vi "Fully Dynamic FPGA Interface Example.vi"() -> ()   [LabVIEW 2010]
uses:
  <vilib>/userDefined/High Color/nirio_resource_hc.ctl
  TypeDefs/Fully Dynamic FPGA Interface TypeDef.ctl
  <vilib>/Utility/sysdir.llb/System Directory Type.ctl
  <userlib>/_FPGA Interface Advanced Tools/FPGA Interface Base/FPGA Interface Base.lvclass
  <userlib>/_FPGA Interface Advanced Tools/FPGA Bitfile Utility/Get Register Map.vi
  <userlib>/_FPGA Interface Advanced Tools/FPGA Bitfile Utility/Get Base Address.vi
  <vilib>/rvi/Utilities/XML/nirviXML_GetValue.vi
  <vilib>/rvi/Utilities/XML/nirviXML_GetValue_String.vi
  <vilib>/rvi/Bitfile/niFpgaReadBitfileXml_VIRegisterMap.vi
  <vilib>/rvi/Utilities/XML/nirviXML_GetValue_U32.vi
  <vilib>/Utility/VariantDataType/GetTypeInfo.vi
  <vilib>/Utility/VariantDataType/GetArrayInfo.vi
  <userlib>/_FPGA Interface Advanced Tools/FPGA Interface Base/FPGA Read By Name - Boolean.vi
  <userlib>/_FPGA Interface Advanced Tools/FPGA Interface Base/FPGA Read By Name - I8.vi
  <userlib>/_FPGA Interface Advanced Tools/FPGA Interface Base/FPGA Read By Name - I16.vi
  <userlib>/_FPGA Interface Advanced Tools/FPGA Interface Base/FPGA Read By Name - I32.vi
  <userlib>/_FPGA Interface Advanced Tools/FPGA Interface Base/FPGA Read By Name - I64.vi
  <userlib>/_FPGA Interface Advanced Tools/FPGA Interface Base/FPGA Read By Name - U8.vi
  <userlib>/_FPGA Interface Advanced Tools/FPGA Interface Base/FPGA Read By Name - U16.vi
  <userlib>/_FPGA Interface Advanced Tools/FPGA Interface Base/FPGA Read By Name - U32.vi
  <userlib>/_FPGA Interface Advanced Tools/FPGA Interface Base/FPGA Read By Name - U64.vi
  <userlib>/_FPGA Interface Advanced Tools/FPGA Interface Base/FPGA Read Array By Name - Boolean.vi
  <userlib>/_FPGA Interface Advanced Tools/FPGA Interface Base/FPGA Read Array By Name - I8.vi
  <userlib>/_FPGA Interface Advanced Tools/FPGA Interface Base/FPGA Read Array By Name - I16.vi
  <userlib>/_FPGA Interface Advanced Tools/FPGA Interface Base/FPGA Read Array By Name - I32.vi
  <userlib>/_FPGA Interface Advanced Tools/FPGA Interface Base/FPGA Read Array By Name - I64.vi
  <userlib>/_FPGA Interface Advanced Tools/FPGA Interface Base/FPGA Read Array By Name - U8.vi
  <userlib>/_FPGA Interface Advanced Tools/FPGA Interface Base/FPGA Read Array By Name - U16.vi
  <userlib>/_FPGA Interface Advanced Tools/FPGA Interface Base/FPGA Read Array By Name - U32.vi
  <userlib>/_FPGA Interface Advanced Tools/FPGA Interface Base/FPGA Read Array By Name - U64.vi
  <userlib>/_FPGA Interface Advanced Tools/FPGA Interface Base/FPGA Write By Name - Boolean.vi
  <userlib>/_FPGA Interface Advanced Tools/FPGA Interface Base/FPGA Write By Name - I8.vi
  <userlib>/_FPGA Interface Advanced Tools/FPGA Interface Base/FPGA Write By Name - I16.vi
  <userlib>/_FPGA Interface Advanced Tools/FPGA Interface Base/FPGA Write By Name - I32.vi
  <userlib>/_FPGA Interface Advanced Tools/FPGA Interface Base/FPGA Write By Name - I64.vi
  <userlib>/_FPGA Interface Advanced Tools/FPGA Interface Base/FPGA Write By Name - U8.vi
  <userlib>/_FPGA Interface Advanced Tools/FPGA Interface Base/FPGA Write By Name - U16.vi
  <userlib>/_FPGA Interface Advanced Tools/FPGA Interface Base/FPGA Write By Name - U32.vi
  <userlib>/_FPGA Interface Advanced Tools/FPGA Interface Base/FPGA Write By Name - U64.vi
  <userlib>/_FPGA Interface Advanced Tools/FPGA Interface Base/FPGA Write Array By Name - Boolean.vi
  <userlib>/_FPGA Interface Advanced Tools/FPGA Interface Base/FPGA Write Array By Name - I8.vi
  <userlib>/_FPGA Interface Advanced Tools/FPGA Interface Base/FPGA Write Array By Name - I16.vi
  <userlib>/_FPGA Interface Advanced Tools/FPGA Interface Base/FPGA Write Array By Name - I32.vi
  <userlib>/_FPGA Interface Advanced Tools/FPGA Interface Base/FPGA Write Array By Name - I64.vi
  <userlib>/_FPGA Interface Advanced Tools/FPGA Interface Base/FPGA Write Array By Name - U8.vi
  <userlib>/_FPGA Interface Advanced Tools/FPGA Interface Base/FPGA Write Array By Name - U16.vi
  <userlib>/_FPGA Interface Advanced Tools/FPGA Interface Base/FPGA Write Array By Name - U32.vi
  <userlib>/_FPGA Interface Advanced Tools/FPGA Interface Base/FPGA Write Array By Name - U64.vi
  <userlib>/_FPGA Interface Advanced Tools/FPGA Bitfile Utility/FPGA Bitfile Utility.lvlib
panel:
  in  "RIO Resource":T1="RIO0"
  out "Boolean Array Read":bool[](array[boolean])
  in  "Boolean Array Write":bool[](array[boolean])
  in  "Numeric Array Write":dbl[](array[numeric])
  out "Numeric Array Read":dbl[](array[numeric])
  in  "Numeric Write":dbl
  out "Numeric Read":dbl
  in  "Boolean Write":bool
  out "Bool Read":bool
  in  "Write":bool
  in  "Read":bool
  in  "Multicolumn Listbox":i32(listbox)
  in  "Stop FPGA":bool
  in  "Run FPGA":bool
  in  "Select Bitfile":bool
  out "Bifile Path":path
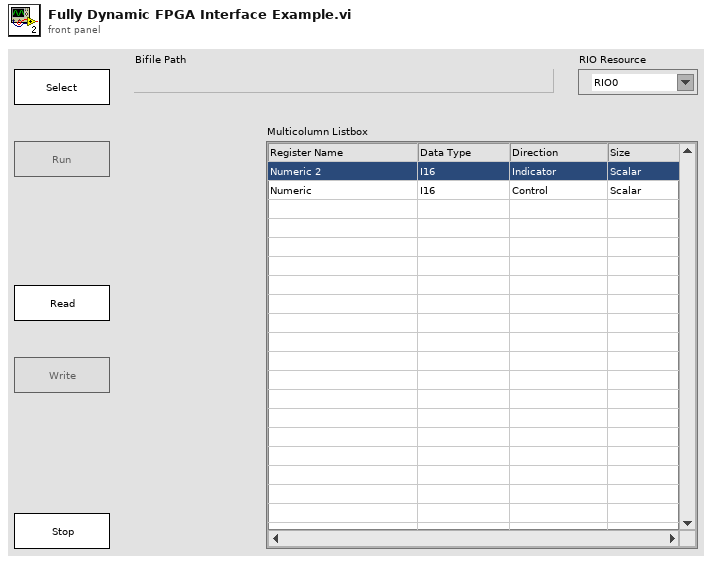
[diagram p1: front panel]
types:
  T1 = typedef "nirio_resource_hc.ctl" = tag
  T2 = typedef "Fully Dynamic FPGA Interface TypeDef.ctl" = enum16{"Idle", "Init", "Read", "Write"}
  T3 = enum8{"Enabled", "Disabled", "Disabled and Grayed Out"}
  T4 = typedef "System Directory Type.ctl" = i32
  T5 = typedef "FPGA Bitfile Utility.lvlib/Control_Indicator Info.ctl" = cluster{"Array?":bool, "Data Type":T6, "Address":u32, "Num Elements":u32, "Name":string}
  T6 = typedef "niFpgaDataTypeControl.ctl" = enum32{"Boolean", "I8", "I16", "I32", "I64", "U8", "U16", "U32", "U64", "FXP", "CustomControl"}
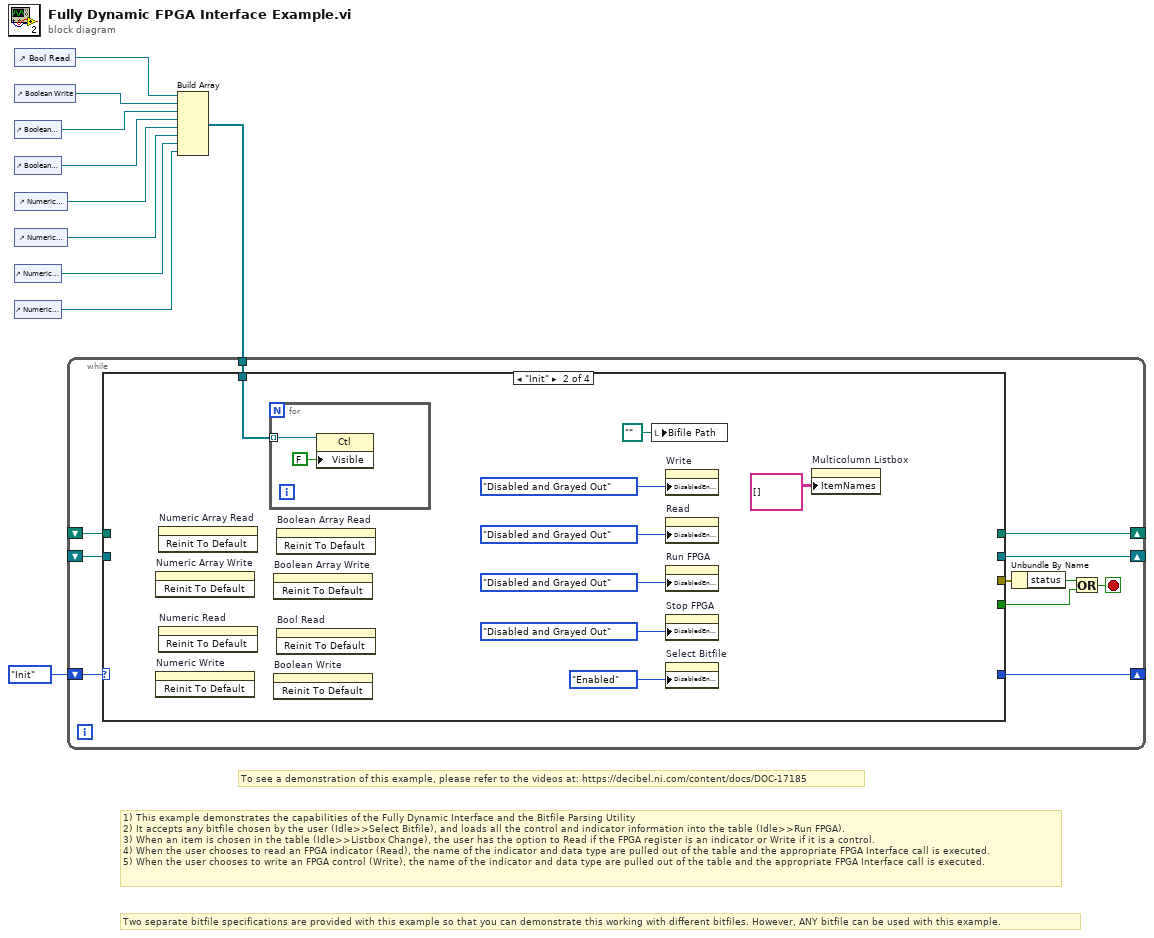
[diagram p0: block diagram]
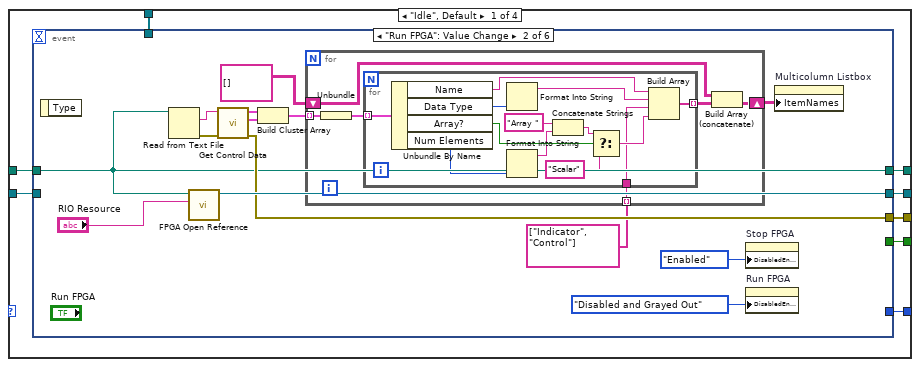
[diagram p2: hidden frame]
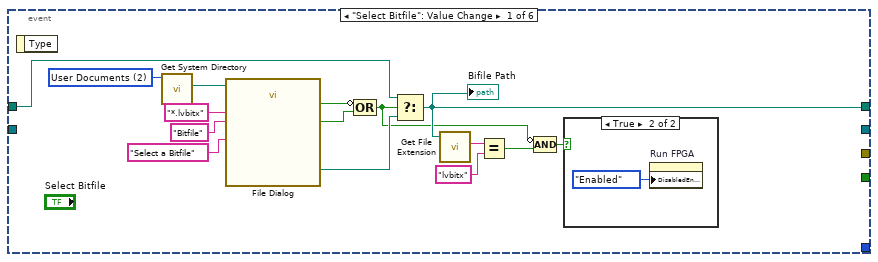
[diagram p3: hidden frame]
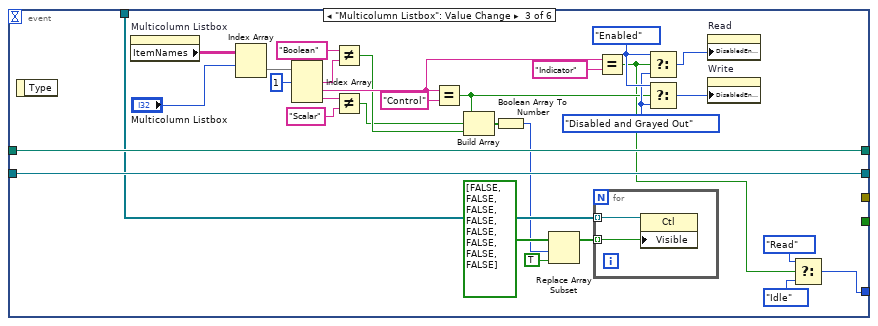
[diagram p5: hidden frame]
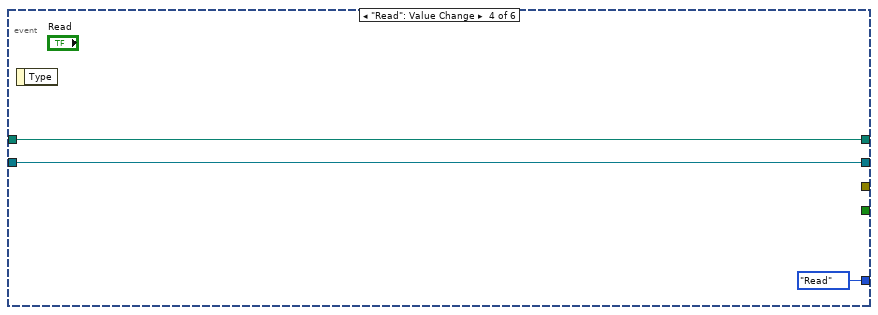
[diagram p6: hidden frame]
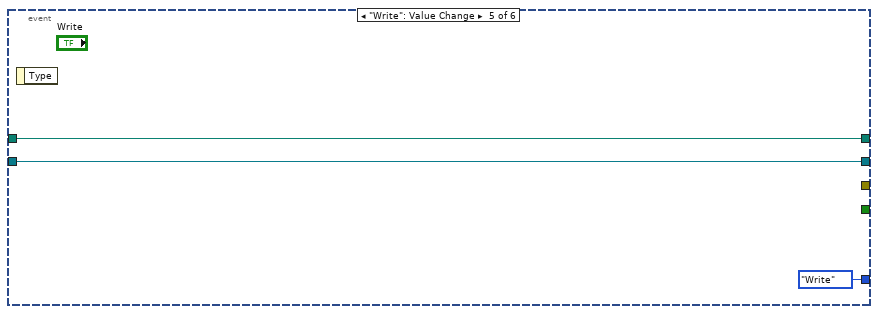
[diagram p7: hidden frame]
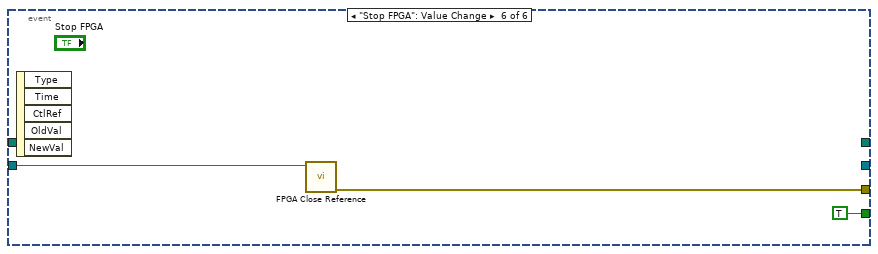
[diagram p8: hidden frame]
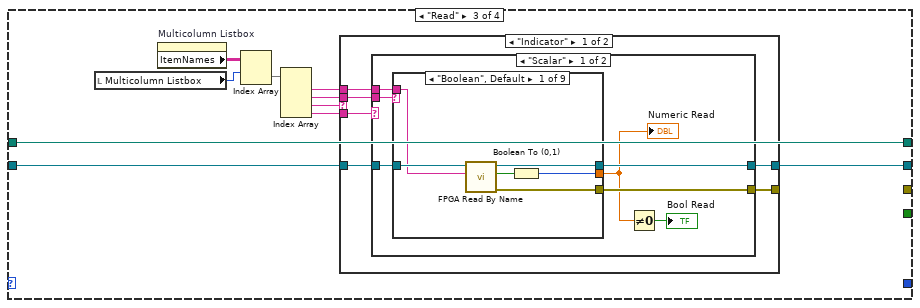
[diagram p9: hidden frame]
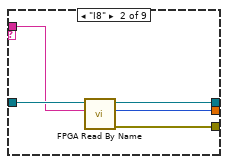
[diagram p10: hidden frame]
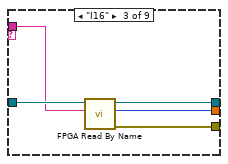
[diagram p11: hidden frame]
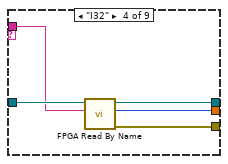
[diagram p12: hidden frame]
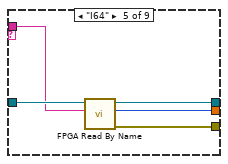
[diagram p13: hidden frame]
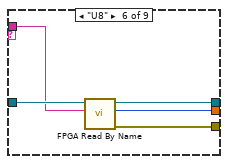
[diagram p14: hidden frame]
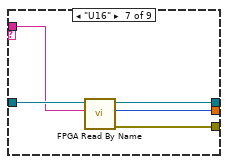
[diagram p15: hidden frame]
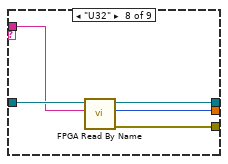
[diagram p16: hidden frame]
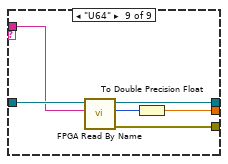
[diagram p17: hidden frame]
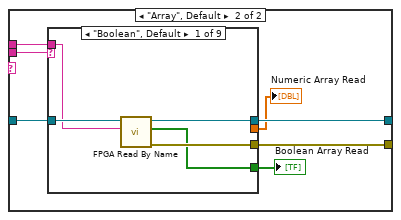
[diagram p18: hidden frame]
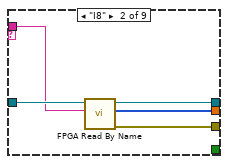
[diagram p19: hidden frame]
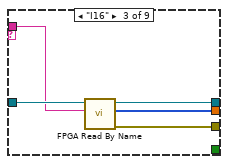
[diagram p20: hidden frame]
diagram:
  # "Two separate bitfile specifications are provided with this example so that you can demonstrate this working with different bitfiles. However, ANY bitfile can be used with this example."
  # "1) This example demonstrates the capabilities of the Fully Dynamic Interface and the Bitfile Parsing Utility\n2) It accepts any bitfile chosen by the user (Idle>>Select Bitfile), and loads all the control and indicator information into the table (Idle>>Run FPGA).\n3) When an item is chosen in the table (Idle>>Listbox Change), the user has the option to Read if the FPGA register is an indicator or Write if it is a control.\n4) When the user chooses to read an FPGA indicator (Read), the name of the indicator and data type are pulled out of the table and the appropriate FPGA Interface call is executed.\n5) When the user chooses to write an FPGA control (Write), the name of the indicator and data type are pulled out of the table and the appropriate FPGA Interface call is executed."
  # "To see a demonstration of this example, please refer to the videos at: https://decibel.ni.com/content/docs/DOC-17185"
  n1 = control-ref of="Bool Read"() -> (w10:refnum<vi>)
  n2 = control-ref of="Boolean Write"() -> (w6:refnum<vi>)
  n3 = control-ref of="Boolean Array Read"() -> (w7:refnum<vi>)
  n4 = control-ref of="Boolean Array Write"() -> (w8:refnum<vi>)
  n5 = control-ref of="Numeric Read"() -> (w5:refnum<vi>)
  n6 = control-ref of="Numeric Write"() -> (w4:refnum<vi>)
  n7 = control-ref of="Numeric Array Read"() -> (w3:refnum<vi>)
  n8 = control-ref of="Numeric Array Write"() -> (w2:refnum<vi>)
  n9 = Build Array(w10, w6, w7, w8, w5, w4, w3, w2) -> (w9:refnum<vi>[])
  n10 = while {
    shift-right: [w21] -> _
    shift-left: _ -> [w20]
    shift-right: [w19] -> _
    shift-left: _ -> [w18]
    tunnel: w9 -> [w14]
    shift-right: [w12] -> _
    shift-left: Fully_Dynamic_FPGA_Interface_TypeDef."Init" -> [w13]
    stop <- w16 stop-if-true
    n11 = case shown="\"Init\"" w13 {
      tunnel: [w29 _ w130 w254] -> w21
      tunnel: w20 -> [w28 _ w130 w254]
      tunnel: [w27 _ w131 w255] -> w19
      tunnel: w18 -> [w26 _ w132 w256]
      tunnel: [w25 _ _ _] -> w17
      tunnel: [w24 _ _ _] -> w15
      tunnel: w14 -> [w23 w120 _ _]
      tunnel: [w22 _ _ _] -> w12
      frame "Idle", Default {
        n12 = event shown="[1] \"Run FPGA\": Value Change" {
          selector: _ -> [_ _ _ _ _ _]
          dyn-events: _ -> [_ _ _ _ _ _]
          timeout: _ -> [_ _ _ _ _ _]
          tunnel: [w35 w55 w99 w112 w114 _] -> w29
          tunnel: w28 -> [w36 w55 w99 w112 w114 _]
          tunnel: [_ w59 w100 w111 w115 _] -> w27
          tunnel: w26 -> [_ _ w100 w111 w115 w119]
          tunnel: [_ w56 _ _ _ w118] -> w25
          tunnel: [_ _ _ _ _ TRUE] -> w24
          tunnel: w23 -> [_ _ w96 _ _ _]
          tunnel: [_ _ w81 Fully_Dynamic_FPGA_Interface_TypeDef."Read" Fully_Dynamic_FPGA_Interface_TypeDef."Write" _] -> w22
          event "Select Bitfile": Value Change {
            w44 = T4 2 items=["User Home"=0, "User Desktop"=1, "User Documents"=2, "User Application Data"=3, "User Preferences"=4, "User Temporary"=5, "Public Documents"=6, "Public Application Data"=7, "Public Preferences"=8, "Public Cache"=13, "System Core Libraries"=9, "System Installed Libraries"=10, "Application Files"=11, "Boot Volume Root"=12] ("system directory type")
            n13 = event-data() -> ()  [unwired: 1 in, 1 out]
            n14 = call <vilib>:"Get System Directory.vi"("system directory type"=w44) -> ("system directory"=w43:path)  [unwired: 10 in]
            n15 = call "File Dialog"("start path"=w43, "prompt"="Select a Bitfile", "pattern (all files)"="*.lvbitx", "pattern label"="Bitfile") -> ("selected path"=w37:path, "exists"=w38:bool, "cancelled"=w39:bool)  [unwired: 8 in, 1 out]
            n16 = Compound Arithmetic op=OR(invert w38, w39) -> (w30:bool)
            n17 = Select(t=w36, s=w30, f=w37) -> (s? t:f=w35:path)
            "Bifile Path" <- w35
            n18 = call <vilib>:"Get File Extension.vi"("file"=w35) -> ("lowercase file extension"=w34:string)  [unwired: 7 in, 3 out]
            n19 = Equal?(x=w34, y="lvbitx") -> (x = y?=w32:bool)
            n20 = Compound Arithmetic op=AND(invert w30, w32) -> (w31:bool)
            n21 = case shown="True" w31 {
              frame False {
              }
              frame True {
                n22 = property on="Run FPGA" class="Bool"("DisabledEnum"=T3."Enabled" ("Disabled")) -> ()  [unwired: 2 in, 2 out]
              }
            }
          }
          event "Run FPGA": Value Change {
            n23 = event-data() -> ()  [unwired: 1 in, 1 out]
            n24 = Read from Text File(file (use dialog)=w55) -> (text=w58:string, error out=w57:errorcluster)  [unwired: 3 in, 2 out]
            n25 = call <userlib>:"FPGA Open Reference.vi"("FPGA Resource"="RIO Resource", "Bitfile Path"=w55) -> ("FPGA Session"=w59:refnum<class "FPGA Interface Base.lvclass">)  [unwired: 8 in, 1 out]
            n26 = call <userlib>:"Get Control Data.vi"("error in (no error)"=w57, "bitfile xml in"=w58) -> ("error out"=w56:errorcluster, "Controls"=w52:T5[], "Indicators"=w54:T5[])  [unwired: 6 in, 1 out]
            n27 = Build Cluster Array(w54, w52) -> (w53:cluster{"Controls":T5[]}[])
            n28 = for {
              tunnel: w53 -> [w65] mode=indexing
              tunnel: string[] ["Indicator", "Control"] -> [w64] mode=indexing
              shift-right: [w63] -> w50
              shift-left: string[][] [] -> [w62]
              n29 = Unbundle(w65) -> ("Controls"=w60:T5[])
              n30 = for {
                tunnel: w60 -> [w78] mode=indexing
                tunnel: [w67] -> w61 mode=indexing
                tunnel: w64 -> [w66]
                n31 = Unbundle By Name(w78) -> ("Name"=w70:string, "Data Type"=w77:T6, "Array?"=w76:bool, "Num Elements"=w75:u32)
                n32 = Format Into String(w77) -> (resulting string=w69:string)  [unwired: 3 in, 1 out]
                n33 = Format Into String(w75) -> (resulting string=w73:string)  [unwired: 3 in, 1 out]
                n34 = Concatenate Strings("Array " ("Name"), w73) -> (w72:string)
                n35 = Select(t=w72, s=w76, f="Scalar" ("Name")) -> (s? t:f=w68:string)
                n36 = Build Array(w70, w69, w66, w68) -> (w67:string[])
              }
              n37 = Build Array (concatenate)(w62, w61) -> (w63:string[][])
            }
            n38 = property on="Stop FPGA" class="Bool"("DisabledEnum"=T3."Enabled" ("Disabled")) -> ()  [unwired: 2 in, 2 out]
            n39 = property on="Run FPGA" class="Bool"("DisabledEnum"=T3."Disabled and Grayed Out" ("Disabled")) -> ()  [unwired: 2 in, 2 out]
            n40 = property on="Multicolumn Listbox" class="MCListbox (strict)"("ItemNames"=w50) -> ()  [unwired: 2 in, 2 out]
          }
          event "Multicolumn Listbox": Value Change {
            w98 = T3."Disabled and Grayed Out" ("Disabled")
            w103 = T3."Enabled" ("Disabled")
            n41 = event-data() -> ()  [unwired: 1 in, 1 out]
            n42 = property on="Multicolumn Listbox" class="MCListbox (strict)"() -> ("ItemNames"=w108:string[][])  [unwired: 2 in, 2 out]
            n43 = Index Array(array=w108, index (row)="Multicolumn Listbox") -> (element=w104:string[])  [unwired: 1 in]
            n44 = Index Array(array=w104, index #1=1 ("index")) -> (element #1=w91:string, element #2=w92:string, element #3=w88:string)  [unwired: 2 in]
            n45 = Not Equal?(x="Boolean", y=w91) -> (x != y?=w89:bool)
            n46 = Not Equal?(x=w88, y="Scalar") -> (x != y?=w84:bool)
            n47 = Equal?(x=w92, y="Control") -> (x = y?=w80:bool)
            n48 = Build Array(w80, w84, w89) -> (w86:bool[])
            n49 = Boolean Array To Number(Boolean array=w86) -> (number=w85:u32)
            n50 = Replace Array Subset(array=bool[] [FALSE, FALSE, FALSE, FALSE, FALSE, FALSE, FALSE, FALSE], new element=TRUE ("new element/subarray"), index=w85) -> (w95:bool[])
            n51 = for {
              tunnel: w96 -> [w110] mode=indexing
              tunnel: w95 -> [w109] mode=indexing
              n52 = property class="Ctl"(reference=w110, "Visible"=w109) -> ()  [unwired: 1 in, 2 out]
            }
            n53 = Equal?(x=w92, y="Indicator") -> (x = y?=w79:bool)
            n54 = Select(t=w103, s=w79, f=w98) -> (s? t:f=w101:T3)
            n55 = Select(t=w103, s=w80, f=w98) -> (s? t:f=w102:T3)
            n56 = property on="Read" class="Bool"("DisabledEnum"=w101) -> ()  [unwired: 2 in, 2 out]
            n57 = property on="Write" class="Bool"("DisabledEnum"=w102) -> ()  [unwired: 2 in, 2 out]
            n58 = Select(t=Fully_Dynamic_FPGA_Interface_TypeDef."Read", s=w79, f=Fully_Dynamic_FPGA_Interface_TypeDef."Idle") -> (s? t:f=w81:T2)
          }
          event "Read": Value Change {
            n59 = event-data() -> ()  [unwired: 1 in, 1 out]
          }
          event "Write": Value Change {
            n60 = event-data() -> ()  [unwired: 1 in, 1 out]
          }
          event "Stop FPGA": Value Change {
            n61 = event-data() -> ()  [unwired: 1 in, 5 out]
            n62 = call-dynamic "FPGA Close Reference.vi"("FPGA Session In"=w119) -> ("error out"=w118:errorcluster)  [unwired: 10 in]
          }
        }
      }
      frame "Init" {
        n63 = invoke on="Numeric Array Write" class="Arr (strict)" method="Reinit To Default"() -> ()  [unwired: 3 in, 3 out]
        n64 = invoke on="Numeric Write" class="DigNum (strict)" method="Reinit To Default"() -> ()  [unwired: 3 in, 3 out]
        n65 = invoke on="Numeric Array Read" class="Arr (strict)" method="Reinit To Default"() -> ()  [unwired: 3 in, 3 out]
        n66 = invoke on="Numeric Read" class="DigNum (strict)" method="Reinit To Default"() -> ()  [unwired: 3 in, 3 out]
        n67 = for {
          tunnel: w120 -> [w129] mode=indexing
          n68 = property class="Ctl"(reference=w129, "Visible"=FALSE) -> ()  [unwired: 1 in, 2 out]
        }
        n69 = invoke on="Boolean Array Write" class="Arr (strict)" method="Reinit To Default"() -> ()  [unwired: 3 in, 3 out]
        n70 = invoke on="Boolean Write" class="Bool (strict)" method="Reinit To Default"() -> ()  [unwired: 3 in, 3 out]
        n71 = invoke on="Boolean Array Read" class="Arr (strict)" method="Reinit To Default"() -> ()  [unwired: 3 in, 3 out]
        n72 = invoke on="Bool Read" class="Bool (strict)" method="Reinit To Default"() -> ()  [unwired: 3 in, 3 out]
        n73 = local write "Bifile Path"(path "" ("Bifile Path")) -> ()
        n74 = property on="Write" class="Bool"("DisabledEnum"=T3."Disabled and Grayed Out" ("Disabled")) -> ()  [unwired: 2 in, 2 out]
        n75 = property on="Read" class="Bool"("DisabledEnum"=T3."Disabled and Grayed Out" ("Disabled")) -> ()  [unwired: 2 in, 2 out]
        n76 = property on="Run FPGA" class="Bool"("DisabledEnum"=T3."Disabled and Grayed Out" ("Disabled")) -> ()  [unwired: 2 in, 2 out]
        n77 = property on="Stop FPGA" class="Bool"("DisabledEnum"=T3."Disabled and Grayed Out" ("Disabled")) -> ()  [unwired: 2 in, 2 out]
        n78 = property on="Select Bitfile" class="Bool"("DisabledEnum"=T3."Enabled" ("Disabled")) -> ()  [unwired: 2 in, 2 out]
        n79 = property on="Multicolumn Listbox" class="MCListbox (strict)"("ItemNames"=string[][] [] ("Item Names")) -> ()  [unwired: 2 in, 2 out]
      }
      frame "Read" {
        n80 = local read "Multicolumn Listbox"() -> (w138:i32)
        n81 = property on="Multicolumn Listbox" class="MCListbox (strict)"() -> ("ItemNames"=w139:string[][])  [unwired: 2 in, 2 out]
        n82 = Index Array(array=w139, index (row)=w138) -> (element=w137:string[])  [unwired: 1 in]
        n83 = Index Array(array=w137) -> (element #1=w135:string, element #2=w134:string, element #3=w136:string, element #4=w133:string)  [unwired: 4 in]
        n84 = case shown="\"Indicator\"" w136 {
          tunnel: w135 -> [w142 _]
          tunnel: w134 -> [w144 _]
          tunnel: w133 -> [w145 _]
          tunnel: w132 -> [w143 w253]
          tunnel: [w141 w253] -> w131
          tunnel: [w140 _] -> _
          frame "Indicator" {
            n85 = case shown="\"Scalar\"" w145 {
              tunnel: w144 -> [w152 w205]
              tunnel: w143 -> [w151 w204]
              tunnel: w142 -> [w150 w206]
              tunnel: [w149 w203] -> w141
              tunnel: [w148 w202] -> w140
              frame "Scalar" {
                n86 = case shown="\"Boolean\", Default" w152 {
                  tunnel: w151 -> [w158 w163 w168 w173 w178 w183 w188 w193 w199]
                  tunnel: w150 -> [w157 w162 w167 w172 w177 w182 w187 w192 w198]
                  tunnel: [w155 w161 w166 w171 w176 w181 w186 w191 w197] -> w149
                  tunnel: [w156 w160 w165 w170 w175 w180 w185 w190 w196] -> w148
                  tunnel: [w153 w159 w164 w169 w174 w179 w184 w189 w194] -> w146
                  frame "Boolean", Default {
                    n87 = call-poly <userlib>:"FPGA Read By Name.vi"("Indicator"=w157, "FPGA Session In"=w158) -> ("error out"=w156:errorcluster, "Value"=w154:bool, "FPGA Session Out"=w155:refnum<class "FPGA Interface Base.lvclass">)  [unwired: 7 in]
                    n88 = Boolean To (0,1)(Boolean=w154) -> (0, 1=w153:i16)
                  }
                  frame "I8" {
                    n89 = call-poly <userlib>:"FPGA Read By Name.vi"("Indicator"=w162, "FPGA Session In"=w163) -> ("error out"=w160:errorcluster, "Value"=w159:i8, "FPGA Session Out"=w161:refnum<class "FPGA Interface Base.lvclass">)  [unwired: 7 in]
                  }
                  frame "I16" {
                    n90 = call-poly <userlib>:"FPGA Read By Name.vi"("Indicator"=w167, "FPGA Session In"=w168) -> ("error out"=w165:errorcluster, "Value"=w164:i16, "FPGA Session Out"=w166:refnum<class "FPGA Interface Base.lvclass">)  [unwired: 7 in]
                  }
                  frame "I32" {
                    n91 = call-poly <userlib>:"FPGA Read By Name.vi"("Indicator"=w172, "FPGA Session In"=w173) -> ("error out"=w170:errorcluster, "Value"=w169:i32, "FPGA Session Out"=w171:refnum<class "FPGA Interface Base.lvclass">)  [unwired: 7 in]
                  }
                  frame "I64" {
                    n92 = call-poly <userlib>:"FPGA Read By Name.vi"("Indicator"=w177, "FPGA Session In"=w178) -> ("error out"=w175:errorcluster, "Value"=w174:i64, "FPGA Session Out"=w176:refnum<class "FPGA Interface Base.lvclass">)  [unwired: 7 in]
                  }
                  frame "U8" {
                    n93 = call-poly <userlib>:"FPGA Read By Name.vi"("Indicator"=w182, "FPGA Session In"=w183) -> ("error out"=w180:errorcluster, "Value"=w179:u8, "FPGA Session Out"=w181:refnum<class "FPGA Interface Base.lvclass">)  [unwired: 7 in]
                  }
                  frame "U16" {
                    n94 = call-poly <userlib>:"FPGA Read By Name.vi"("Indicator"=w187, "FPGA Session In"=w188) -> ("error out"=w185:errorcluster, "Value"=w184:u16, "FPGA Session Out"=w186:refnum<class "FPGA Interface Base.lvclass">)  [unwired: 7 in]
                  }
                  frame "U32" {
                    n95 = call-poly <userlib>:"FPGA Read By Name.vi"("Indicator"=w192, "FPGA Session In"=w193) -> ("error out"=w190:errorcluster, "Value"=w189:u32, "FPGA Session Out"=w191:refnum<class "FPGA Interface Base.lvclass">)  [unwired: 7 in]
                  }
                  frame "U64" {
                    n96 = call-poly <userlib>:"FPGA Read By Name.vi"("Indicator"=w198, "FPGA Session In"=w199) -> ("error out"=w196:errorcluster, "Value"=w195:u64, "FPGA Session Out"=w197:refnum<class "FPGA Interface Base.lvclass">)  [unwired: 7 in]
                    n97 = To Double Precision Float(number=w195) -> (double precision float=w194:dbl)
                  }
                }
                "Numeric Read" <- w146
                n98 = Not Equal To 0?(x=w146) -> (x != 0?=→"Bool Read":bool)
              }
              frame "Array", Default {
                n99 = case shown="\"Boolean\", Default" w205 {
                  tunnel: w204 -> [w211 w216 w221 w226 w231 w236 w241 w246 w252]
                  tunnel: w206 -> [w210 w215 w220 w225 w230 w235 w240 w245 w251]
                  tunnel: [w208 w214 w219 w224 w229 w234 w239 w244 w250] -> w203
                  tunnel: [w209 w213 w218 w223 w228 w233 w238 w243 w249] -> w202
                  tunnel: [_ w212 w217 w222 w227 w232 w237 w242 w247] -> w200
                  tunnel: [w207 _ _ _ _ _ _ _ _] -> w201
                  frame "Boolean", Default {
                    n100 = call-poly <userlib>:"FPGA Read By Name.vi"("Indicator"=w210, "FPGA Session In"=w211) -> ("error out"=w209:errorcluster, "Array"=w207:bool[], "FPGA Session Out"=w208:refnum<class "FPGA Interface Base.lvclass">)  [unwired: 7 in]
                  }
                  frame "I8" {
                    n101 = call-poly <userlib>:"FPGA Read By Name.vi"("Indicator"=w215, "FPGA Session In"=w216) -> ("error out"=w213:errorcluster, "Array"=w212:i8[], "FPGA Session Out"=w214:refnum<class "FPGA Interface Base.lvclass">)  [unwired: 7 in]
                  }
                  frame "I16" {
                    n102 = call-poly <userlib>:"FPGA Read By Name.vi"("Indicator"=w220, "FPGA Session In"=w221) -> ("error out"=w218:errorcluster, "Array"=w217:i16[], "FPGA Session Out"=w219:refnum<class "FPGA Interface Base.lvclass">)  [unwired: 7 in]
                  }
                  frame "I32" {
                    n103 = call-poly <userlib>:"FPGA Read By Name.vi"("Indicator"=w225, "FPGA Session In"=w226) -> ("error out"=w223:errorcluster, "Array"=w222:i32[], "FPGA Session Out"=w224:refnum<class "FPGA Interface Base.lvclass">)  [unwired: 7 in]
                  }
                  frame "I64" {
                    n104 = call-poly <userlib>:"FPGA Read By Name.vi"("Indicator"=w230, "FPGA Session In"=w231) -> ("error out"=w228:errorcluster, "Array"=w227:i64[], "FPGA Session Out"=w229:refnum<class "FPGA Interface Base.lvclass">)  [unwired: 7 in]
                  }
                  frame "U8" {
                    n105 = call-poly <userlib>:"FPGA Read By Name.vi"("Indicator"=w235, "FPGA Session In"=w236) -> ("error out"=w233:errorcluster, "Array"=w232:u8[], "FPGA Session Out"=w234:refnum<class "FPGA Interface Base.lvclass">)  [unwired: 7 in]
                  }
                  frame "U16" {
                    n106 = call-poly <userlib>:"FPGA Read By Name.vi"("Indicator"=w240, "FPGA Session In"=w241) -> ("error out"=w238:errorcluster, "Array"=w237:u16[], "FPGA Session Out"=w239:refnum<class "FPGA Interface Base.lvclass">)  [unwired: 7 in]
                  }
                  frame "U32" {
                    n107 = call-poly <userlib>:"FPGA Read By Name.vi"("Indicator"=w245, "FPGA Session In"=w246) -> ("error out"=w243:errorcluster, "Array"=w242:u32[], "FPGA Session Out"=w244:refnum<class "FPGA Interface Base.lvclass">)  [unwired: 7 in]
                  }
                  frame "U64" {
                    n108 = call-poly <userlib>:"FPGA Read By Name.vi"("Indicator"=w251, "FPGA Session In"=w252) -> ("error out"=w249:errorcluster, "Array"=w248:u64[], "FPGA Session Out"=w250:refnum<class "FPGA Interface Base.lvclass">)  [unwired: 7 in]
                    n109 = To Double Precision Float(number=w248) -> (double precision float=w247:dbl[])
                  }
                }
                "Boolean Array Read" <- w201
                "Numeric Array Read" <- w200
              }
            }
          }
          frame "Control", Default {
          }
        }
      }
      frame "Write" {
        n110 = local read "Multicolumn Listbox"() -> (w262:i32)
        n111 = property on="Multicolumn Listbox" class="MCListbox (strict)"() -> ("ItemNames"=w263:string[][])  [unwired: 2 in, 2 out]
        n112 = Index Array(array=w263, index (row)=w262) -> (element=w261:string[])  [unwired: 1 in]
        n113 = Index Array(array=w261) -> (element #1=w259:string, element #2=w258:string, element #3=w260:string, element #4=w257:string)  [unwired: 4 in]
        n114 = case shown="\"Control\"" w260 {
          tunnel: w259 -> [w266 _]
          tunnel: w258 -> [w268 _]
          tunnel: w257 -> [w269 _]
          tunnel: w256 -> [w267 w374]
          tunnel: [w265 w374] -> w255
          tunnel: [w264 _] -> _
          frame "Control" {
            n115 = case shown="\"Array\", Default" w269 {
              tunnel: w268 -> [w276 w327]
              tunnel: w267 -> [w275 w326]
              tunnel: w266 -> [w274 w328]
              tunnel: [w273 w325] -> w265
              tunnel: [w272 w324] -> w264
              frame "Scalar" {
                n116 = case shown="\"Boolean\", Default" w276 {
                  tunnel: w275 -> [w281 w286 w291 w296 w301 w306 w311 w316 w321]
                  tunnel: w274 -> [w280 w285 w290 w295 w300 w305 w310 w315 w320]
                  tunnel: [w278 w283 w288 w293 w298 w303 w308 w313 w318] -> w273
                  tunnel: [w279 w284 w289 w294 w299 w304 w309 w314 w319] -> w272
                  tunnel: "Boolean Write" -> [w277 _ _ _ _ _ _ _ _]
                  tunnel: "Numeric Write" -> [_ w282 w287 w292 w297 w302 w307 w312 w317]
                  frame "Boolean", Default {
                    n117 = call-poly <userlib>:"FPGA Write By Name.vi"("Value"=w277, "Control"=w280, "FPGA Session In"=w281) -> ("error out"=w279:errorcluster, "FPGA Session Out"=w278:refnum<class "FPGA Interface Base.lvclass">)  [unwired: 7 in]
                  }
                  frame "I8" {
                    n118 = call-poly <userlib>:"FPGA Write By Name.vi"("Value"=w282, "Control"=w285, "FPGA Session In"=w286) -> ("error out"=w284:errorcluster, "FPGA Session Out"=w283:refnum<class "FPGA Interface Base.lvclass">)  [unwired: 7 in]
                  }
                  frame "I16" {
                    n119 = call-poly <userlib>:"FPGA Write By Name.vi"("Value"=w287, "Control"=w290, "FPGA Session In"=w291) -> ("error out"=w289:errorcluster, "FPGA Session Out"=w288:refnum<class "FPGA Interface Base.lvclass">)  [unwired: 7 in]
                  }
                  frame "I32" {
                    n120 = call-poly <userlib>:"FPGA Write By Name.vi"("Value"=w292, "Control"=w295, "FPGA Session In"=w296) -> ("error out"=w294:errorcluster, "FPGA Session Out"=w293:refnum<class "FPGA Interface Base.lvclass">)  [unwired: 7 in]
                  }
                  frame "I64" {
                    n121 = call-poly <userlib>:"FPGA Write By Name.vi"("Value"=w297, "Control"=w300, "FPGA Session In"=w301) -> ("error out"=w299:errorcluster, "FPGA Session Out"=w298:refnum<class "FPGA Interface Base.lvclass">)  [unwired: 7 in]
                  }
                  frame "U8" {
                    n122 = call-poly <userlib>:"FPGA Write By Name.vi"("Value"=w302, "Control"=w305, "FPGA Session In"=w306) -> ("error out"=w304:errorcluster, "FPGA Session Out"=w303:refnum<class "FPGA Interface Base.lvclass">)  [unwired: 7 in]
                  }
                  frame "U16" {
                    n123 = call-poly <userlib>:"FPGA Write By Name.vi"("Value"=w307, "Control"=w310, "FPGA Session In"=w311) -> ("error out"=w309:errorcluster, "FPGA Session Out"=w308:refnum<class "FPGA Interface Base.lvclass">)  [unwired: 7 in]
                  }
                  frame "U32" {
                    n124 = call-poly <userlib>:"FPGA Write By Name.vi"("Value"=w312, "Control"=w315, "FPGA Session In"=w316) -> ("error out"=w314:errorcluster, "FPGA Session Out"=w313:refnum<class "FPGA Interface Base.lvclass">)  [unwired: 7 in]
                  }
                  frame "U64" {
                    n125 = call-poly <userlib>:"FPGA Write By Name.vi"("Value"=w317, "Control"=w320, "FPGA Session In"=w321) -> ("error out"=w319:errorcluster, "FPGA Session Out"=w318:refnum<class "FPGA Interface Base.lvclass">)  [unwired: 7 in]
                  }
                }
              }
              frame "Array", Default {
                n126 = case shown="\"Boolean\", Default" w327 {
                  tunnel: w326 -> [w333 w338 w343 w348 w353 w358 w363 w368 w373]
                  tunnel: w328 -> [w332 w337 w342 w347 w352 w357 w362 w367 w372]
                  tunnel: [w330 w336 w341 w346 w351 w356 w361 w366 w371] -> w325
                  tunnel: [w331 w335 w340 w345 w350 w355 w360 w365 w370] -> w324
                  tunnel: "Numeric Array Write" -> [_ w334 w339 w344 w349 w354 w359 w364 w369]
                  tunnel: "Boolean Array Write" -> [w329 _ _ _ _ _ _ _ _]
                  frame "Boolean", Default {
                    n127 = call-poly <userlib>:"FPGA Write By Name.vi"("Array"=w329, "Control"=w332, "FPGA Session In"=w333) -> ("error out"=w331:errorcluster, "FPGA Session Out"=w330:refnum<class "FPGA Interface Base.lvclass">)  [unwired: 7 in]
                  }
                  frame "I8" {
                    n128 = call-poly <userlib>:"FPGA Write By Name.vi"("Array"=w334, "Control"=w337, "FPGA Session In"=w338) -> ("error out"=w335:errorcluster, "FPGA Session Out"=w336:refnum<class "FPGA Interface Base.lvclass">)  [unwired: 7 in]
                  }
                  frame "I16" {
                    n129 = call-poly <userlib>:"FPGA Write By Name.vi"("Array"=w339, "Control"=w342, "FPGA Session In"=w343) -> ("error out"=w340:errorcluster, "FPGA Session Out"=w341:refnum<class "FPGA Interface Base.lvclass">)  [unwired: 7 in]
                  }
                  frame "I32" {
                    n130 = call-poly <userlib>:"FPGA Write By Name.vi"("Array"=w344, "Control"=w347, "FPGA Session In"=w348) -> ("error out"=w345:errorcluster, "FPGA Session Out"=w346:refnum<class "FPGA Interface Base.lvclass">)  [unwired: 7 in]
                  }
                  frame "I64" {
                    n131 = call-poly <userlib>:"FPGA Write By Name.vi"("Array"=w349, "Control"=w352, "FPGA Session In"=w353) -> ("error out"=w350:errorcluster, "FPGA Session Out"=w351:refnum<class "FPGA Interface Base.lvclass">)  [unwired: 7 in]
                  }
                  frame "U8" {
                    n132 = call-poly <userlib>:"FPGA Write By Name.vi"("Array"=w354, "Control"=w357, "FPGA Session In"=w358) -> ("error out"=w355:errorcluster, "FPGA Session Out"=w356:refnum<class "FPGA Interface Base.lvclass">)  [unwired: 7 in]
                  }
                  frame "U16" {
                    n133 = call-poly <userlib>:"FPGA Write By Name.vi"("Array"=w359, "Control"=w362, "FPGA Session In"=w363) -> ("error out"=w360:errorcluster, "FPGA Session Out"=w361:refnum<class "FPGA Interface Base.lvclass">)  [unwired: 7 in]
                  }
                  frame "U32" {
                    n134 = call-poly <userlib>:"FPGA Write By Name.vi"("Array"=w364, "Control"=w367, "FPGA Session In"=w368) -> ("error out"=w365:errorcluster, "FPGA Session Out"=w366:refnum<class "FPGA Interface Base.lvclass">)  [unwired: 7 in]
                  }
                  frame "U64" {
                    n135 = call-poly <userlib>:"FPGA Write By Name.vi"("Array"=w369, "Control"=w372, "FPGA Session In"=w373) -> ("error out"=w370:errorcluster, "FPGA Session Out"=w371:refnum<class "FPGA Interface Base.lvclass">)  [unwired: 7 in]
                  }
                }
              }
            }
          }
          frame "Indicator", Default {
          }
        }
      }
    }
    n136 = Unbundle By Name(w17) -> ("status"=w11:bool)
    n137 = Or(x=w11, y=w15) -> (x .or. y?=w16:bool)
  }
